vi "SIMPLE.vi"() -> ()   [LabVIEW 2016]
uses:
  <vilib>/Instr/_visa.llb/VISA Set IO Buffer Mask.ctl
  <vilib>/Utility/miscctls.llb/LVPointTypeDef.ctl
  GEN_2.lvlib
  <vilib>/Instr/_visa.llb/VISA Configure Serial Port (Instr).vi
  GEN2_Instructions.ctl
panel:
  out "ERROR":u8
  in  "repeat":bool
  out "x-y":dbl(graph)
  out "write buffer":string
  out "read buffer":string
  in  "Instruction":T1 format="%02x" items=["PING"=1, "READ_STAT"=2, "WRITE_STAT"=3, "READ_CONFIG"=4, "WRITE_CONFIG"=5, "SAVE_CONFIG"=6, "SET_POSI"=8, "BULK_STAT"=18]
  in  "ID":u8 format="%x"
  in  "write":bool
  in  "parameter":string="ÿÿ\u0000\u0002\u0001ü"
  in  "Baud rate":u32=8000000
  in  "Com port":refnum<visa-resource-name>="COM10"
  in  "stop":bool
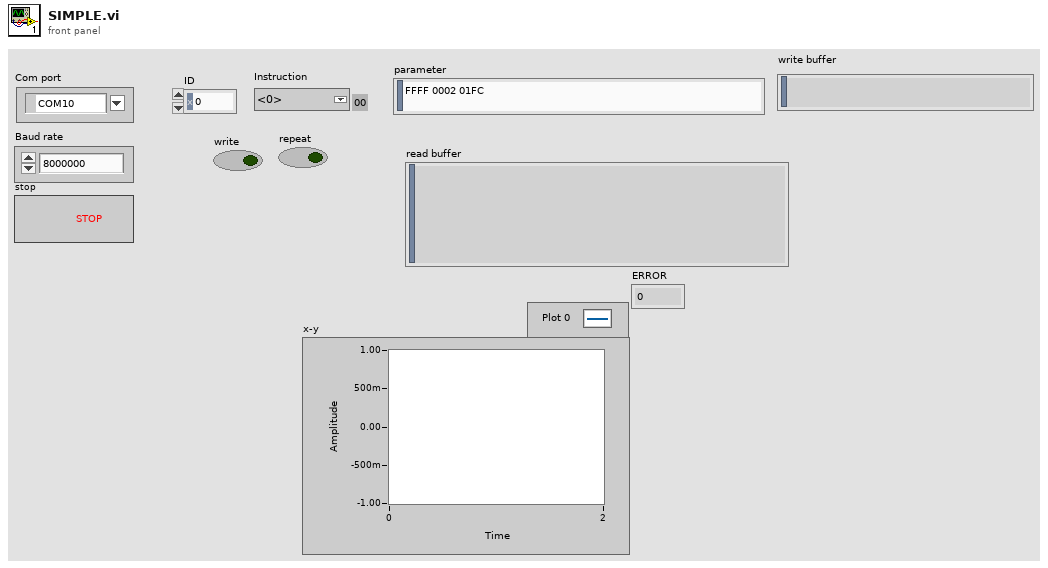
[diagram p1: front panel]
types:
  T1 = typedef "GEN_2.lvlib/GEN2_Instructions.ctl" = u8
  T2 = typedef "LVPointTypeDef.ctl" = cluster{"Horizontal":i16, "Vertical":i16}
  T3 = typedef "VISA Set IO Buffer Mask.ctl" = u16
  T4 = cluster{"ID":u8, "ERROR":u8, "ChechSumError?":bool, "Data":string}
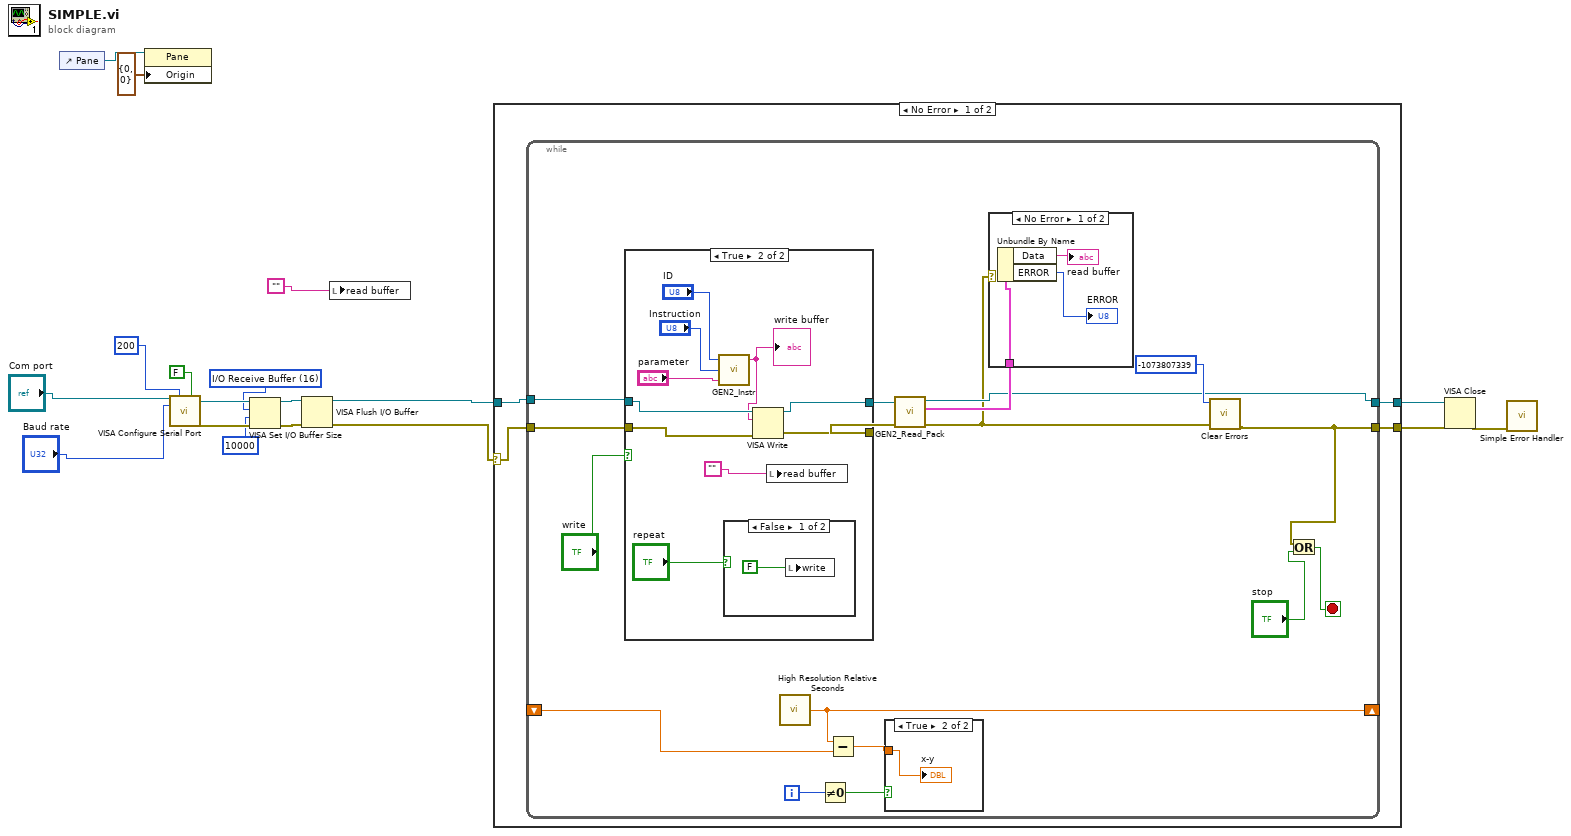
[diagram p0: block diagram]
diagram:
  w10 = T3 16 items=["I/O Receive Buffer"=16, "I/O Transmit Buffer"=32, "I/O Receive and Transmit Buffer"=48] ("Mask")
  n1 = control-ref of="Pane"() -> (w5:refnum<vi>)
  n2 = property class="Pane"(reference=w5, "Origin"=T2 {"Horizontal"=0, "Vertical"=0}) -> ()  [unwired: 1 in, 2 out]
  n3 = call-poly "VISA Configure Serial Port"("VISA resource name"="Com port", "timeout (10sec)"=u32 200, "Enable Termination\nChar (T)"=FALSE ("Enable Termination\nChar (T)"), "baud rate (9600)"="Baud rate") -> ("VISA resource name out"=w11:refnum<visa-resource-name>, "error out"=w14:errorcluster)  [unwired: 10 in]
  n4 = VISA Set I/O Buffer Size(VISA resource name=w11, mask (16)=w10, size (4096)=u32 10000, error in (no error)=w14) -> (VISA resource name out=w12:refnum<visa-resource-name>, error out=w13:errorcluster)
  n5 = VISA Flush I/O Buffer(VISA resource name=w12, error in (no error)=w13) -> (VISA resource name out=w1:refnum<visa-resource-name>, error out=w2:errorcluster)  [unwired: 1 in]
  n6 = local write "read buffer"("") -> ()
  n7 = case shown="No Error" w2 {
    selector: w2 -> [w19 w57]
    tunnel: [w22 w57] -> w18
    tunnel: w1 -> [w21 w58]
    tunnel: [w20 w58] -> w16
    frame No Error {
      n8 = while {
        tunnel: w21 -> [w35]
        tunnel: w19 -> [w34]
        tunnel: [w30] -> w20
        tunnel: [w29] -> w22
        shift-right: [w27] -> _
        shift-left: _ -> [w26]
        i -> [w24]
        stop <- w38 stop-if-true
        n9 = case shown="True" "write" {
          tunnel: w34 -> [w45 w55]
          tunnel: w35 -> [w44 w54]
          tunnel: [w44 w53] -> w32
          tunnel: [w45 w52] -> w33
          frame False {
          }
          frame True {
            n10 = call "GEN2_Instr.vi"("Parameter"="parameter", "Instruction"="Instruction", "ID"="ID") -> ("Output"=w48:string)  [unwired: 2 in]
            "write buffer" <- w48
            n11 = case shown="False" "repeat" {
              frame False {
                n12 = local write "write"(FALSE ("Clear Screen")) -> ()
              }
              frame True {
              }
            }
            n13 = VISA Write(VISA resource name=w54, write buffer=w48, error in (no error)=w55) -> (VISA resource name out=w53:refnum<visa-resource-name>, error out=w52:errorcluster)  [unwired: 1 out]
            n14 = local write "read buffer"("") -> ()
          }
        }
        n15 = call <vilib>:"High Resolution Relative Seconds.vi"() -> ("relative seconds"=w27:dbl)
        n16 = Not Equal To 0?(x=w24) -> (x != 0?=w23:bool)
        n17 = Subtract(x=w27, y=w26) -> (x-y=w25:dbl)
        n18 = case shown="True" w23 {
          tunnel: w25 -> [_ w40]
          frame False {
          }
          frame True {
            "x-y" <- w40
          }
        }
        n19 = call "GEN2_Read_Pack.vi"("error in (no error)"=w33, "VISA Refnum in"=w32) -> ("error out"=w28:errorcluster, "Pack data"=w31:T4, "VISA Refnum out"=w30:refnum<visa-resource-name>)  [unwired: 7 in]
        n20 = case shown="No Error" w28 {
          tunnel: w31 -> [w43 _]
          frame No Error {
            n21 = Unbundle By Name(w43) -> ("Data"=→"read buffer":string, "ERROR"=→"ERROR":u8)
          }
          frame Error {
          }
        }
        n22 = call <vilib>:"Clear Errors.vi"("error in (no error)"=w28, "specific error code to clear (0: all)"=-1073807339) -> ("error out"=w29:errorcluster)  [unwired: 4 in, 1 out]
        n23 = Or(x=w29, y="stop") -> (x .or. y?=w38:bool)
      }
    }
    frame Error {
    }
  }
  n24 = VISA Close(VISA resource name=w16, error in (no error)=w18) -> (error out=w8:errorcluster)
  n25 = call <vilib>:"Simple Error Handler.vi"("error in (no error)"=w8) -> ()  [unwired: 4 in, 5 out]
